vi "Pixy I2C.vi"() -> ()   [LabVIEW 2016]
doc: "This example shows how to communicate and interpret data for a PIXY camera."
uses:
  <vilib>/Rock Robotics/SystemInterfaces/i2clib/i2c_bus.ctl
  <vilib>/Rock Robotics/WPI/SPI/WPI_SPIMode.ctl
panel:
  in  "CC Objects":bool=TRUE
  in  "Objects":bool=TRUE
  out "CC Objects":T1(array[cluster])
  out "Totals":T2
  in  "Image Brightness":u8(slide)=80 scale=0.0..255.0
  out "ms between frames":u32(graph)
  in  "Shape Colors":u32[](array[colorbox])=[16748288, 16746709, 1244948]
  in  "LED Color":cluster{"Red":u8, "Green":u8, "Blue":u8} {"Blue" scale=0.0..255.0; "Green" scale=0.0..255.0; "Red" scale=0.0..255.0}
  out "Picture":picture
  out "Objects":T3(array[cluster])
  # "Top left of roboRIO"
  # "Back of PIXY"
  # "1  2\n 3  4\n 5  6\n 7  8\n 9 10"
  # "I2C cable\nPIXY      roboRIO\nPin 5 ----- SCL\nPin 9 ----- SDA\nPin 10 --- GND"
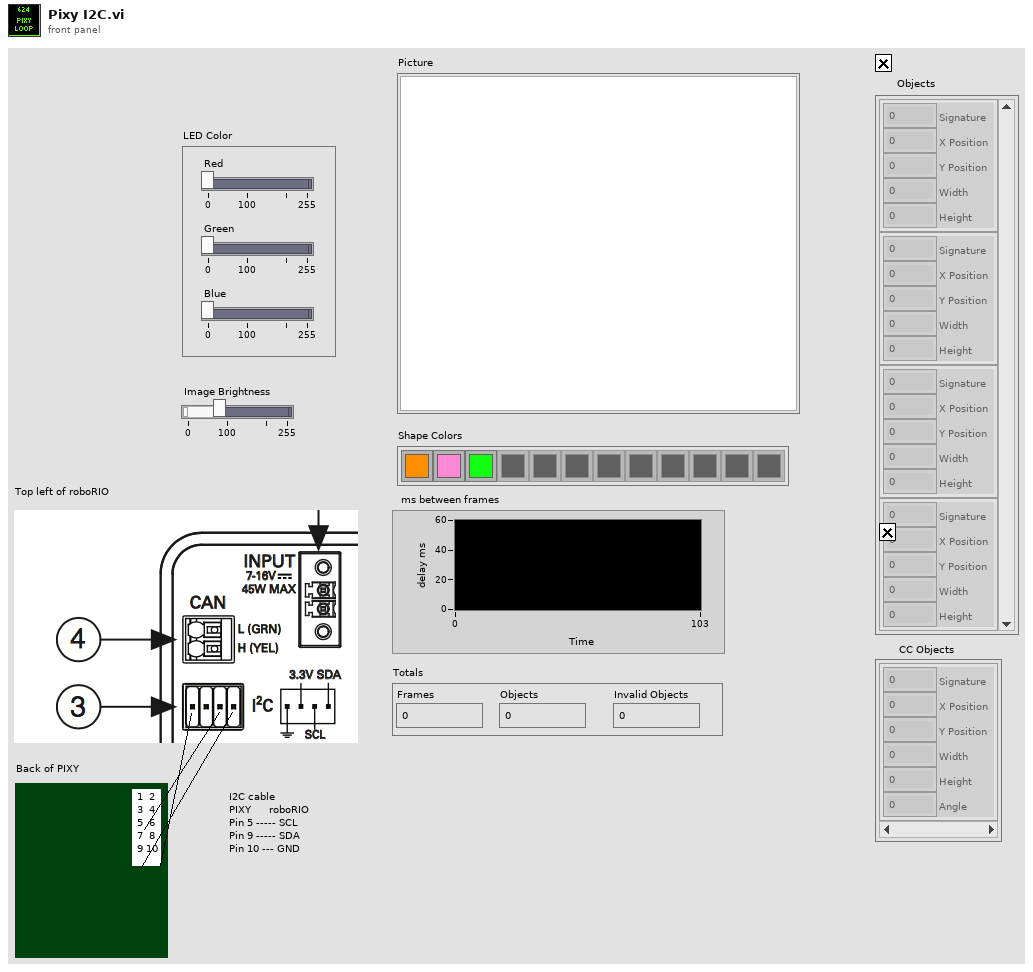
[diagram p1: front panel]
types:
  T1 = cluster{"Signature":u16, "X Position":u16, "Y Position":u16, "Width":u16, "Height":u16, "Angle":i16}[]
  T2 = cluster{"Frames":u32, "Objects":u32, "Invalid Objects":i32}
  T3 = cluster{"Signature":u16, "X Position":u16, "Y Position":u16, "Width":u16, "Height":u16}[]
  T4 = typedef "i2c_bus.ctl" = enum16{"I2C On-Board", "I2C MXP", "Invalid"}
  T5 = enum16{"Read Objects", "Write LED Color", "Write Brightness", "Write Objects", "Read Settings"}
  T6 = typedef "WPI_SPIMode.ctl" = enum16{"Mode 0 (Clk Idle Low,Sample on Leading)", "Mode 1 (Clk Idle Low,Sample on Trailing)", "Mode 2 (Clk Idle High,Sample on Leading)", "Mode 3 (Clk Idle High,Sample on Trailing)"}
  T7 = typedef "WPI_SPIDevRef.ctl" = cluster{"DevStatus":errorcluster, "Handle":i32, "SPI Bus":T8}
  T8 = typedef "spi_bus.ctl" = enum16{"SPI On-Board, CS0", "SPI On-Board, CS1", "SPI On-Board, CS2", "SPI On-Board, CS3", "SPI MXP", "Invalid"}
  T9 = typedef "WPI_I2CDevRef.ctl" = cluster{"DevStatus":errorcluster, "Device Address":u8, "Handle":i32, "I2C Bus":T4}
  T10 = cluster{"Signature":u16, "X Position":u16, "Y Position":u16, "Width":u16, "Height":u16}
  T11 = cluster{"Signature":u16, "X Position":u16, "Y Position":u16, "Width":u16, "Height":u16, "Angle":i16}
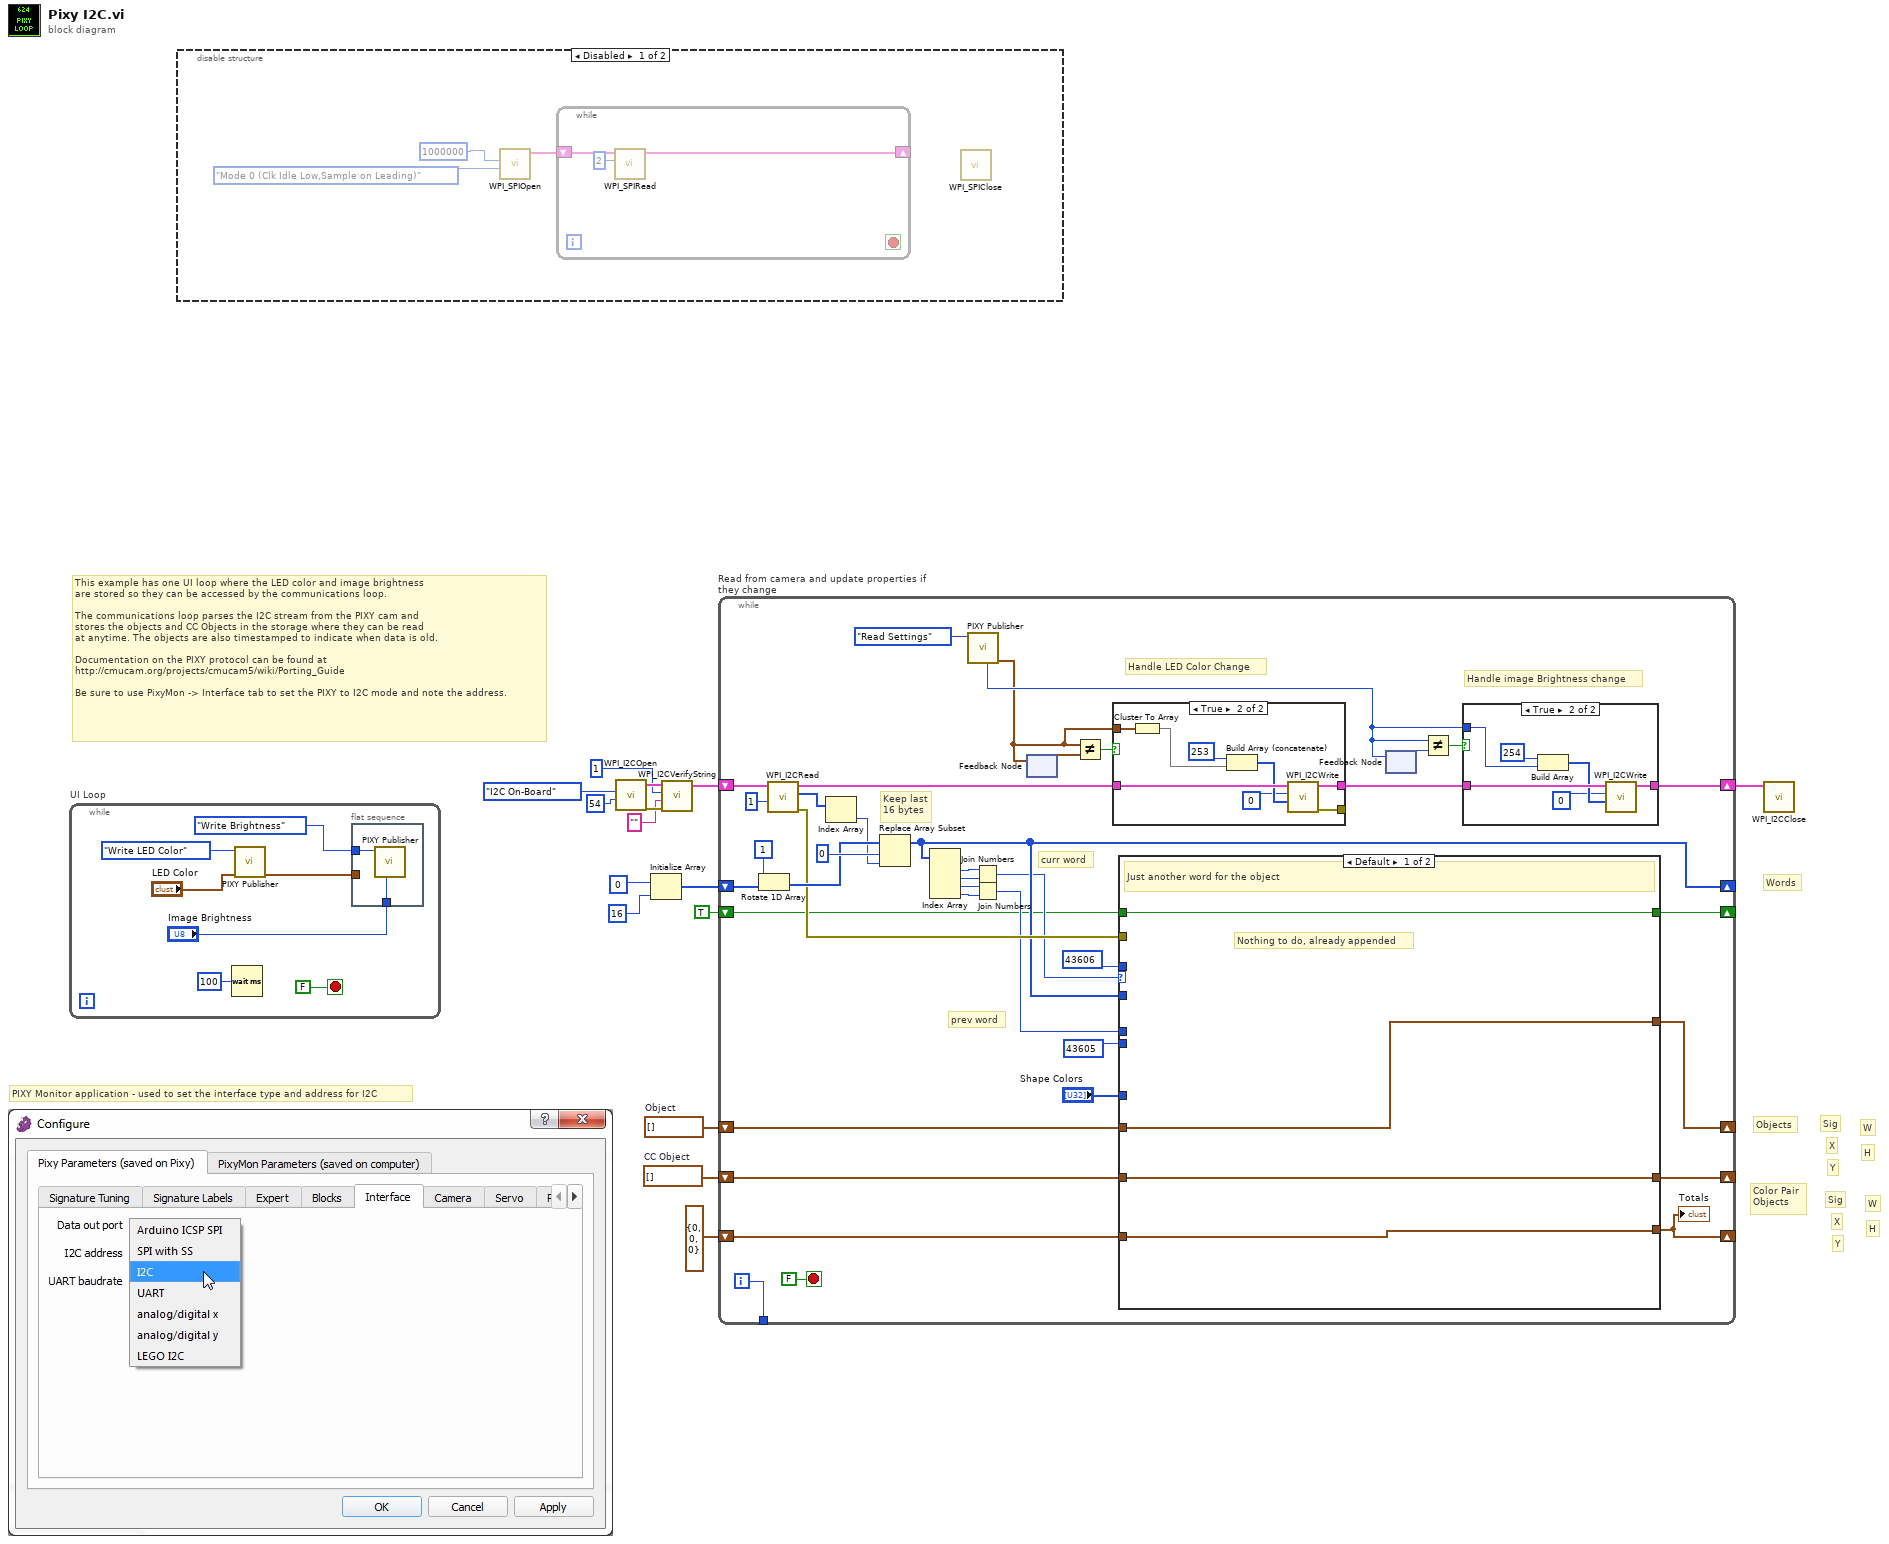
[diagram p0: block diagram]
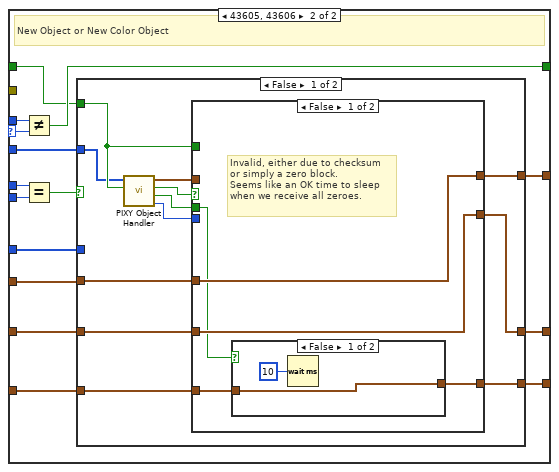
[diagram p2: hidden frame]
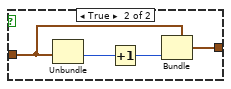
[diagram p3: hidden frame]
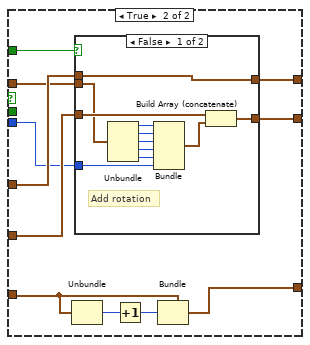
[diagram p4: hidden frame]
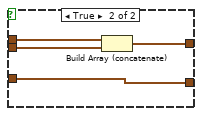
[diagram p5: hidden frame]
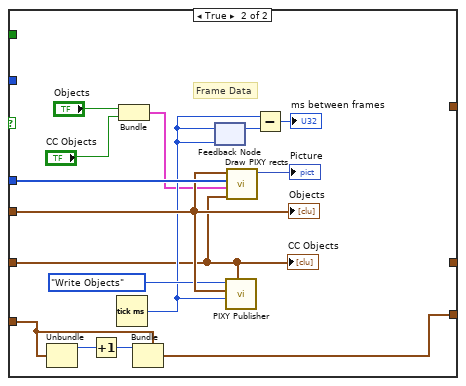
[diagram p6: hidden frame]
diagram:
  w10 = T1 []  # CC Object
  w11 = T3 []  # Object
  # "PIXY Monitor application - used to set the interface type and address for I2C"
  # "This example has one UI loop where the LED color and image brightness\nare stored so they can be accessed by the communications loop.\n\nThe communications loop parses the I2C stream from the PIXY cam and\nstores the objects and CC Objects in the storage where they can be read\nat anytime. The objects are also timestamped to indicate when data is old.\n\nDocumentation on the PIXY protocol can be found at\nhttp://cmucam.org/projects/cmucam5/wiki/Porting_Guide\n\nBe sure to use PixyMon -> Interface tab to set the PIXY to I2C mode and note the address."
  # "H"
  # "W"
  # "Y"
  # "X"
  # "Sig"
  # "Color Pair\nObjects"
  # "H"
  # "W"
  # "Y"
  # "X"
  # "Sig"
  # "Objects"
  # "Words"
  n1 = while "UI Loop" {
    stop <- FALSE stop-if-true
    n2 = Wait (ms)(milliseconds to wait=u32 100) -> ()  [unwired: 1 out]
    n3 = call "PIXY Publisher.vi"("Color"="LED Color", "Operation"=T5."Write LED Color") -> ("Color Out"=w17:cluster{"Red":u8, "Green":u8, "Blue":u8})  [unwired: 5 in, 4 out]
    n4 = flat-sequence {
      tunnel: T5."Write Brightness" ("Operation") -> [w24]
      tunnel: "Image Brightness" -> [w23]
      tunnel: w17 -> [_]
      frame #0 {
        n5 = call "PIXY Publisher.vi"("Brightness"=w23, "Operation"=w24) -> ()  [unwired: 5 in, 5 out]
      }
    }
  }
  n6 = disable-structure shown="Disabled" {
    frame Disabled {
      n7 = call <vilib>:"WPI_SPIOpen.vi"("Mode (3)"=WPI_SPIMode."Mode 0 (Clk Idle Low,Sample on Leading)", "Clock Rate (Hz)"=1000000) -> ("SPIDevRef"=w25:T7)  [unwired: 4 in, 5 out]
      n8 = while {
        shift-right: [w28] -> _
        shift-left: w25 -> [w30]
        stop <- _ stop-if-true
        n9 = call <vilib>:"WPI_SPIRead.vi"("Num to Read"=2, "SPIDevRef"=w30) -> ("SPIDevRef"=w28:T7)  [unwired: 7 in, 2 out]
      }
      n10 = call <vilib>:"WPI_SPIClose.vi"() -> ()  [unwired: 11 in, 1 out]
    }
    frame Enabled {
    }
  }
  n11 = call <vilib>:"WPI_I2COpen.vi"("Device Address"=u8 54, "I2C Bus"=i2c_bus."I2C On-Board") -> ("error out"=w4:errorcluster, "I2CDevRef"=w5:T9)  [unwired: 8 in]
  n12 = Initialize Array(u8 0 ("Num to Read"), 16 ("Num to Read")) -> (w12:u8[])
  n13 = call <vilib>:"WPI_I2CVerifyString.vi"("error in (no error)"=w4, "Expected"="", "Register Address"=u8 1, "I2CDevRef"=w5) -> ("I2CDevRef"=w1:T9)  [unwired: 6 in, 1 out]
  n14 = while "Read from camera and update properties if they change" {
    shift-right: [w55] -> w15
    shift-left: w1 -> [w69]
    shift-right: [w37] -> _
    shift-left: w12 -> [w60]
    shift-right: [w63] -> _
    shift-left: w11 -> [w64]
    tunnel: [w62] -> _
    shift-right: [w53] -> _
    shift-left: w10 -> [w54]
    shift-right: [w33] -> _
    shift-left: T2 {"Frames"=0, "Objects"=0, "Invalid Objects"=0} ("Totals") -> [w34]
    shift-right: [w31] -> _
    shift-left: TRUE -> [w32]
    i -> [w62]
    stop <- FALSE stop-if-true
    # "curr word"
    # "Handle image Brightness change"
    # "Handle LED Color Change"
    # "prev word"
    # "Keep last\n16 bytes"
    n15 = Rotate 1D Array(1:w60, 2:1 ("Num to Read")) -> (0:w61:u8[])
    n16 = call <vilib>:"WPI_I2CRead.vi"("I2CBytesToRead"=u8 1, "I2CDevRef"=w69) -> ("error out"=w44:errorcluster, "Data Out"=w67:u8[], "I2CDevRef"=w59:T9)  [unwired: 7 in]
    n17 = Index Array(array=w67) -> (element=w43:u8)  [unwired: 1 in]
    n18 = Replace Array Subset(array=w61, new element=w43, index=0 ("Num to Read")) -> (w37:u8[])
    n19 = Index Array(array=w37) -> (element #1=w42:u8, element #2=w41:u8, element #3=w40:u8, element #4=w39:u8)  [unwired: 4 in]
    n20 = call "PIXY Publisher.vi"("Operation"=T5."Read Settings") -> ("Color Out"=w50:cluster{"Red":u8, "Green":u8, "Blue":u8}, "Brightness Out"=w51:u8)  [unwired: 6 in, 3 out]
    n21 = Join Numbers(hi=w42, lo=w41) -> ((hi.lo)=w36:u16)
    n22 = Join Numbers(hi=w40, lo=w39) -> ((hi.lo)=w38:u16)
    n23 = feedback #1() -> (w58:cluster{"Red":u8, "Green":u8, "Blue":u8})  [unwired: 1 in]
    n24 = feedback-in #1(w50) -> ()
    n25 = Not Equal?(x=w50, y=w58) -> (x != y?=w57:bool)
    n26 = case shown="True" w57 {
      tunnel: w59 -> [w160 w168]
      tunnel: [w160 w167] -> w56
      tunnel: w50 -> [_ w166]
      tunnel: [_ w162] -> _
      frame False {
      }
      frame True {
        n27 = Cluster To Array(cluster=w166) -> (array=w165:u8[])
        n28 = Build Array (concatenate)(u8 253 ("Num to Read"), w165) -> (w164:u8[])
        n29 = call <vilib>:"WPI_I2CWrite.vi"("I2CDataToSend"=w164, "I2CRegister"=0 ("Num to Read"), "I2CDevRef"=w168) -> ("error out"=w162:errorcluster, "I2CDevRef"=w167:T9)  [unwired: 7 in]
      }
    }
    n30 = case shown="Default" w36 {
      selector: w36 -> [_ w83]
      tunnel: w38 -> [_ w88]
      tunnel: u16 43605 ("Num to Read") -> [_ w87]
      tunnel: w64 -> [w73 w86]
      tunnel: [w73 w85] -> w63
      tunnel: w37 -> [_ w79]
      tunnel: u16 43606 ("Num to Read") -> [_ w82]
      tunnel: w54 -> [w72 w81]
      tunnel: [w72 w80] -> w53
      tunnel: w44 -> [_ _]
      tunnel: "Shape Colors" -> [_ w78]
      tunnel: w34 -> [w71 w77]
      tunnel: [w71 w76] -> w33
      tunnel: w32 -> [w70 w74]
      tunnel: [w70 w75] -> w31
      frame Default {
        # "Nothing to do, already appended"
        # "Just another word for the object"
      }
      frame 43605, 43606 {
        # "New Object or New Color Object"
        n31 = Not Equal?(x=w82, y=w83) -> (x != y?=w75:bool)
        n32 = Equal?(x=w88, y=w87) -> (x = y?=w84:bool)
        n33 = case shown="False" w84 {
          tunnel: w86 -> [w100 w148]
          tunnel: [w99 _] -> w85
          tunnel: w78 -> [_ w150]
          tunnel: w81 -> [w98 w141]
          tunnel: w74 -> [w93 _]
          tunnel: [w97 _] -> w80
          tunnel: w79 -> [w91 _]
          tunnel: w77 -> [w90 w145]
          tunnel: [w89 w144] -> w76
          frame False {
            n34 = call "PIXY Object Handler.vi"("Normal Object"=w93, "Accumulated Words"=w91) -> ("Angle"=w92:i16, "CheckSum Error"=w94:bool, "Valid"=w95:bool, "Object"=w96:T10)  [unwired: 6 in]
            n35 = case shown="False" w95 {
              tunnel: w100 -> [w105 w122]
              tunnel: [w105 w121] -> w99
              tunnel: w98 -> [w104 w120]
              tunnel: w93 -> [_ w119]
              tunnel: [w104 w118] -> w97
              tunnel: w96 -> [_ w117]
              tunnel: w94 -> [w103 _]
              tunnel: w92 -> [_ w116]
              tunnel: w90 -> [w102 w115]
              tunnel: [w101 w114] -> w89
              frame False {
                # "Invalid, either due to checksum\nor simply a zero block.\nSeems like an OK time to sleep\nwhen we receive all zeroes."
                n36 = case shown="False" w103 {
                  tunnel: w102 -> [w107 w109]
                  tunnel: [w107 w111] -> w101
                  frame False {
                    n37 = Wait (ms)(milliseconds to wait=u32 10) -> ()  [unwired: 1 out]
                  }
                  frame True {
                    n38 = Unbundle(w109) -> ("Invalid Objects"=w110:i32)  [unwired: 2 out]
                    n39 = Increment(x=w110) -> (x+1=w108:i32)
                    n40 = Bundle(cluster=w109, "Invalid Objects"=w108) -> (w111:T2)  [unwired: 2 in]
                  }
                }
              }
              frame True {
                n41 = Unbundle(w115) -> ("Objects"=w113:u32)  [unwired: 2 out]
                n42 = case shown="False" w119 {
                  tunnel: w117 -> [w127 w137]
                  tunnel: w122 -> [w133 w136]
                  tunnel: [w133 w135] -> w121
                  tunnel: w120 -> [w132 w134]
                  tunnel: [w131 w134] -> w118
                  tunnel: w116 -> [w123 _]
                  frame False {
                    # "Add rotation"
                    n43 = Unbundle(w127) -> ("Signature"=w129:u16, "X Position"=w128:u16, "Y Position"=w126:u16, "Width"=w125:u16, "Height"=w124:u16)
                    n44 = Bundle("Signature"=w129, "X Position"=w128, "Y Position"=w126, "Width"=w125, "Height"=w124, "Angle"=w123) -> (w130:T11)  [unwired: 1 in]
                    n45 = Build Array (concatenate)(w132, w130) -> (w131:T1)
                  }
                  frame True {
                    n46 = Build Array (concatenate)(w136, w137) -> (w135:T3)
                  }
                }
                n47 = Increment(x=w113) -> (x+1=w112:u32)
                n48 = Bundle(cluster=w115, "Objects"=w112) -> (w114:T2)  [unwired: 2 in]
              }
            }
          }
          frame True {
            # "Frame Data"
            n49 = Unbundle(w145) -> ("Frames"=w143:u32)  [unwired: 2 out]
            n50 = Increment(x=w143) -> (x+1=w142:u32)
            n51 = Tick Count (ms)() -> (millisecond timer value=w146:u32)
            n52 = Bundle("Objects"="Objects", "CC Objects"="CC Objects") -> (w140:cluster{"Objects":bool, "CC Objects":bool})  [unwired: 1 in]
            n53 = Bundle(cluster=w145, "Frames"=w142) -> (w144:T2)  [unwired: 2 in]
            n54 = feedback #2(w146) -> (w152:u32)
            n55 = feedback-in #2(w146) -> ()
            n56 = call "PIXY Publisher.vi"("Color Combo Object"=w141, "TimeStamp in"=w146, "Object"=w148, "Operation"=T5."Write Objects") -> ()  [unwired: 3 in, 5 out]
            n57 = call "Draw PIXY rects.vi"("CC Objects"=w141, "Draw Options"=w140, "Colors"=w150, "Object"=w148) -> ("Picture"=→"Picture":picture)  [unwired: 7 in]
            n58 = Subtract(x=w146, y=w152) -> (x-y=→"ms between frames":u32)
            "Objects" <- w148
            "CC Objects" <- w141
          }
        }
      }
    }
    "Totals" <- w33
    n59 = feedback #3() -> (w49:u8)  [unwired: 1 in]
    n60 = feedback-in #3(w51) -> ()
    n61 = Not Equal?(x=w51, y=w49) -> (x != y?=w48:bool)
    n62 = case shown="True" w48 {
      tunnel: w56 -> [w153 w159]
      tunnel: [w153 w158] -> w55
      tunnel: w51 -> [_ w154]
      frame False {
      }
      frame True {
        n63 = Build Array(u8 254 ("Num to Read"), w154) -> (w156:u8[])
        n64 = call <vilib>:"WPI_I2CWrite.vi"("I2CDataToSend"=w156, "I2CRegister"=0 ("Num to Read"), "I2CDevRef"=w159) -> ("I2CDevRef"=w158:T9)  [unwired: 7 in, 1 out]
      }
    }
  }
  n65 = call <vilib>:"WPI_I2CClose.vi"("I2CDevRef"=w15) -> ()  [unwired: 10 in, 1 out]
